vi "Create From Structure Reference.vi"(8 "error in (no error)":errorcluster, 10 "Structure":refnum<vi>) -> (0 "error out":errorcluster, 3 "CSM-Helper.lvclass":refnum<class "CSM-Helper.lvclass">)   [LabVIEW 2020, in "CSM-Helper.lvclass"]
uses:
  CSM-Helper.lvclass
  CSM-Helper.lvclass/CSM-Helper.ctl
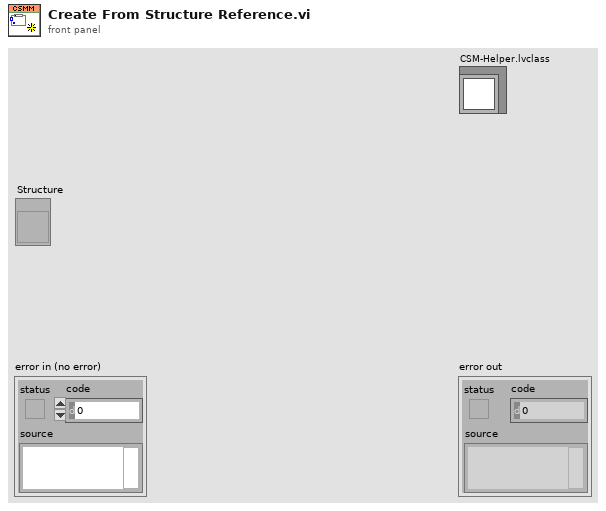
[diagram p1: front panel]
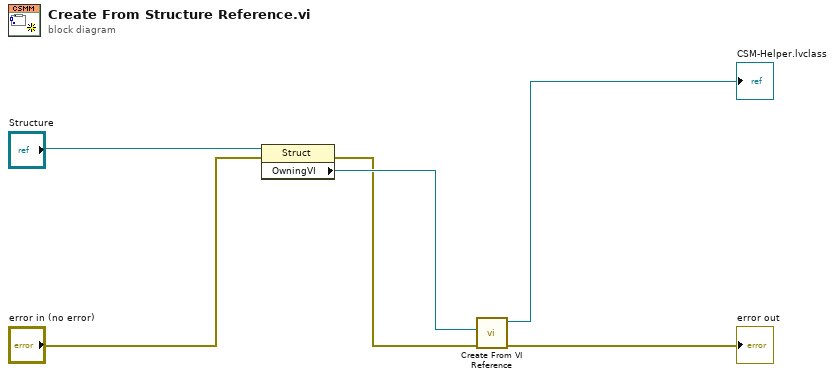
[diagram p0: block diagram]
diagram:
  n1 = property class="Struct"(reference="Structure", error in="error in (no error)") -> (error out=w1:errorcluster, "OwningVI"=w5:refnum<vi>)  [unwired: 1 out]
  n2 = call "Create From VI Reference.vi"("error in (no error)"=w1, "VI"=w5) -> ("error out"=→"error out":errorcluster, "CSM-Helper.lvclass"=→"CSM-Helper.lvclass":refnum<class "CSM-Helper.lvclass">)  [unwired: 8 in]
